vi "NS_ReadProperty.vi"(8 "Error In":errorcluster, 11 "object in":refnum<class "NativeSubTemplate.lvclass">) -> (0 "Error Out":errorcluster, 2 "property":bool, 3 "object out":refnum<class "NativeSubTemplate.lvclass">)   [LabVIEW 2020, in "NativeSubTemplate.lvclass"]
uses:
  <resource>/Framework/Providers/Open_GDS/ClassProviders/Provider_LvNativeClass/Templates/NativeSubTemplate/NativeSubTemplate.lvclass
  <resource>/Framework/Providers/Open_GDS/ClassProviders/Provider_LvNativeClass/Templates/NativeSubTemplate/NativeSubTemplate.lvclass/NativeSubTemplate.ctl
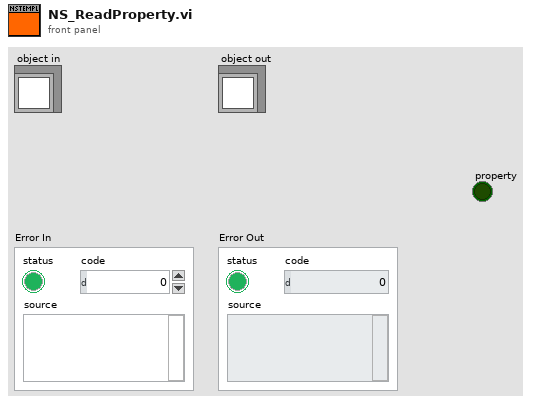
[diagram p1: front panel]
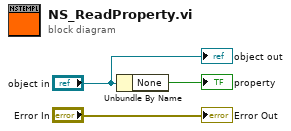
[diagram p0: block diagram]
diagram:
  n1 = Unbundle By Name("object in") -> ("None"=→"property":bool)
  "Error Out" <- "Error In"
  "object out" <- "object in"
